vi "Read Yield Counts.vi"(8 "error in (no error)":errorcluster, 11 "Master in":refnum<class "Master.lvclass">) -> (0 "error out":errorcluster, 3 "Master out":refnum<class "Master.lvclass">)   [LabVIEW 2014, in "Master.lvclass"]
uses:
  Master/Master.lvclass
  Master/Master.lvclass/Master.ctl
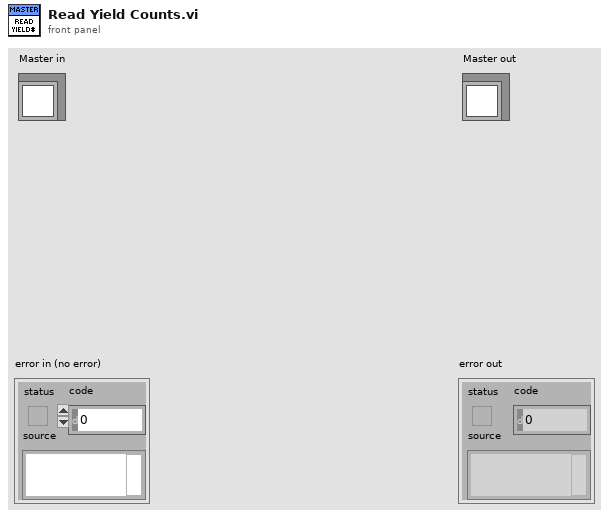
[diagram p1: front panel]
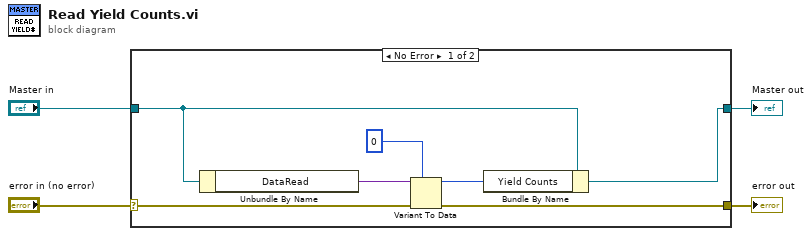
[diagram p0: block diagram]
diagram:
  n1 = case shown="No Error" "error in (no error)" {
    selector: "error in (no error)" -> [w8 w13]
    tunnel: [w7 w13] -> w3
    tunnel: [w9 w12] -> w1
    tunnel: "Master in" -> [w10 w12]
    frame No Error {
      n2 = Unbundle By Name(w10) -> ("DataRead"=w11:variant)
      n3 = Variant To Data(error in=w8, type=0, Variant=w11) -> (data=w6:i32, error out=w7:errorcluster)
      n4 = Bundle By Name(cluster=w10, "Yield Counts"=w6) -> (w9:refnum<class "Master.lvclass">)
    }
    frame Error {
    }
  }
  "error out" <- w3
  "Master out" <- w1
